vi "Unregister for Events.vi"(8 "error in (no error)":errorcluster, 10 "Event Registration Refnum":refnum<event-registration>, 11 "Helper Loop in":refnum<class "Helper Loop.lvclass">) -> (0 "error out":errorcluster, 3 "Helper Loop out":refnum<class "Helper Loop.lvclass">)   [LabVIEW 2024, in "Helper Loop.lvlib" / "Helper Loop.lvclass"]
uses:
  Helper Loop.lvclass
  Helper Loop.lvclass/Helper Loop.ctl
  user events.ctl
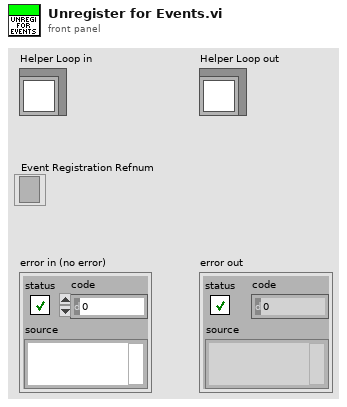
[diagram p1: front panel]
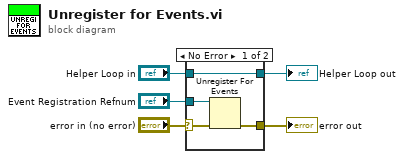
[diagram p0: block diagram]
diagram:
  n1 = case shown="No Error" "error in (no error)" {
    selector: "error in (no error)" -> [w8 w11]
    tunnel: [w7 w11] -> w4
    tunnel: [w9 w10] -> w2
    tunnel: "Helper Loop in" -> [w9 w10]
    tunnel: "Event Registration Refnum" -> [w6 _]
    frame No Error {
      n2 = Unregister For Events(event registration refnum=w6, error in=w8) -> (error out=w7:errorcluster)
    }
    frame Error {
    }
  }
  "error out" <- w4
  "Helper Loop out" <- w2
